vi "Helper.vi"() -> ()   [LabVIEW 2012]
panel:
  in  "Строка поиска":string
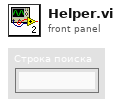
[diagram p1: front panel]
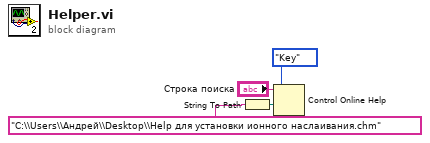
[diagram p0: block diagram]
diagram:
  n1 = String To Path(string="C:\\Users\\Андрей\\Desktop\\Help для установки ионного наслаивания.chm") -> (path=w3:path)
  n2 = Control Online Help(2:w3, 3:"Строка поиска", 4:enum16{"Contents", "Key", "Close"}."Key" ("Operation")) -> ()  [unwired: 1 in, 1 out]
